vi "FTW-Collection-AddOrReplace-String.vi"(0 "Collection":refnum<class "FTW-Collection.lvclass">, 5 "Key":string, 7 "Value":string, 11 "error in":errorcluster) -> (4 "Collection out":refnum<class "FTW-Collection.lvclass">, 6 "Replaced?":bool, 15 "error out":errorcluster)   [LabVIEW 2012, in "FTW-Collection.lvclass"]
uses:
  FTW-Collection.lvclass
panel:
  # "Inputs"
  # "Outputs"
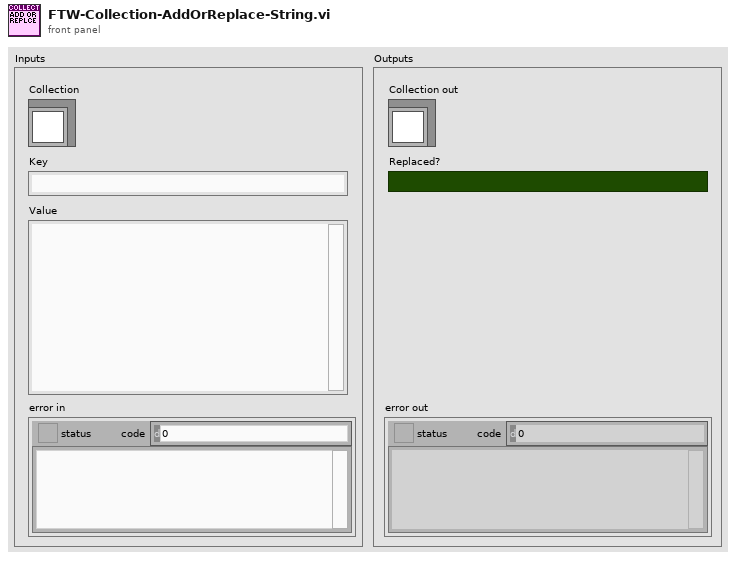
[diagram p1: front panel]
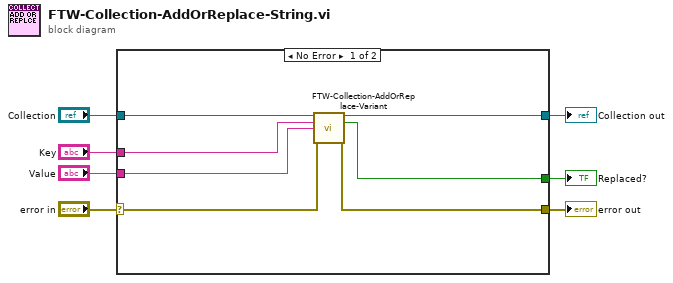
[diagram p0: block diagram]
diagram:
  n1 = case shown="No Error" "error in" {
    selector: "error in" -> [w12 w16]
    tunnel: [w11 w16] -> w7
    tunnel: [w8 _] -> w5
    tunnel: "Collection" -> [w14 w15]
    tunnel: "Key" -> [w10 _]
    tunnel: [w13 w15] -> w2
    tunnel: "Value" -> [w9 _]
    frame No Error {
      n2 = call "FTW-Collection-AddOrReplace-Variant.vi"("Collection"=w14, "Key"=w10, "Value"=w9, "error in"=w12) -> ("Collection out"=w13:refnum<class "FTW-Collection.lvclass">, "Replaced?"=w8:bool, "error out"=w11:errorcluster)  [unwired: 9 in]
    }
    frame Error {
    }
  }
  "error out" <- w7
  "Replaced?" <- w5
  "Collection out" <- w2
